vi "SmartMotor Wait (Command).vi"(0 "reference in":refnum<class "SmartMotor.lvclass">, 5 "error in (no error)":errorcluster) -> (14 "reference out":refnum<class "SmartMotor.lvclass">, 19 "error out":errorcluster)   [LabVIEW 2017, in "SmartMotor.lvclass"]
uses:
  SmartMotor.lvclass
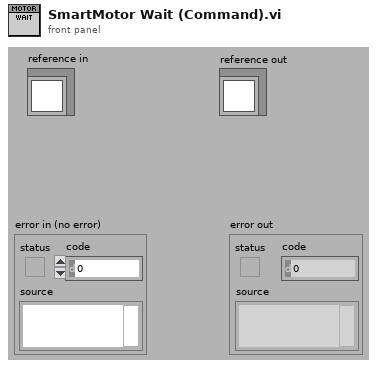
[diagram p1: front panel]
types:
  T1 = typedef "SmartMotor.lvclass/ObjectAttributes.ctl" = cluster{"SmartMotor Chain VISA Resource":refnum<visa-resource-name>, "SmartMotor Chain Address":i16, "Motor Absolute Position":i32, "Motor Relative Position":i32, "Motor Torque":i32, "Motor Voltage":i32, "Screwdriver Engaged":bool, "Screwdriver Torque Limit":i32, "Torque Monitor On/Off Status":bool, "Torque Monitor VI Reference":refnum<vi>, "Absolute Motor Torque (Filtered)":dbl, "SmartMotor Status":T2, "SmartMotor Error":T3}
  T2 = typedef "SmartMotor.lvclass/SmartMotor Status.ctl" = enum8{"Stopped", "Moving"}
  T3 = typedef "SmartMotor.lvclass/SmartMotor Error.ctl" = enum8{"None", "Read Error", "Low Voltage"}
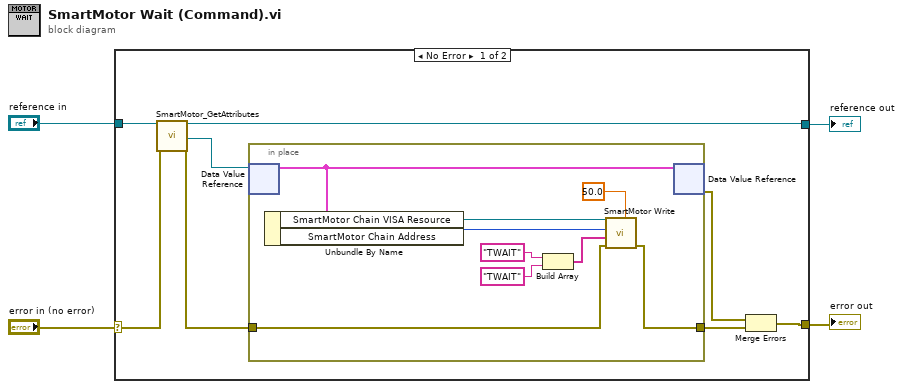
[diagram p0: block diagram]
diagram:
  n1 = case shown="No Error" "error in (no error)" {
    selector: "error in (no error)" -> [w11 w23]
    tunnel: [w8 w23] -> w3
    tunnel: [w9 w22] -> w1
    tunnel: "reference in" -> [w12 w22]
    frame No Error {
      n2 = call "SmartMotor_GetAttributes.vi"("reference in"=w12, "error in (no error)"=w11) -> ("reference out"=w9:refnum<class "SmartMotor.lvclass">, "DataRef"=w7:refnum<data-value>, "error out"=w6:errorcluster)  [unwired: 14 in, 1 out]
      n3 = in-place {
        in-place-border: w6 -> [w18]
        in-place-border: [w17] -> w5
        n4 = in-place-dvr #1(w7) -> (w16:T1)  [unwired: 1 out]
        n5 = Unbundle By Name(w16) -> ("SmartMotor Chain VISA Resource"=w20:refnum<visa-resource-name>, "SmartMotor Chain Address"=w13:i16)
        n6 = Build Array("TWAIT" ("string"), "TWAIT") -> (w21:string[])
        n7 = call "SmartMotor Write.vi"("VISA resource IN"=w20, "Motor Number"=w13, "Motor Command Array"=w21, "Error In"=w18, "Wait Between Writes (ms)"=50.0) -> ("Error Out"=w17:errorcluster)  [unwired: 2 in, 2 out]
        n8 = in-place-dvr #1(w16) -> (w10:errorcluster)  [unwired: 1 out]
      }
      n9 = Merge Errors(w10, w5) -> (w8:errorcluster)
    }
    frame Error {
    }
  }
  "error out" <- w3
  "reference out" <- w1
